vi "Read Application Settings.vi"(8 "error in":errorcluster, 11 "Controller in":refnum<class "Controller.lvclass">) -> (0 "error out":errorcluster, 2 "Application Settings":T4={"Storage Settings"={"Primary Path"=path "", "Backup Storage?"=FALSE, "Backup Path"=path "", "Component Name Prefix"="", "Image Format"=enum."<Select>"}, "PLC Settings"={"Port"="", "BaudRate"=9600, "Wakeup Signal Address "=0, "Acquisiton Address"=0, "Acknowledgement Address"=0, "Sleep Address"=0}, "Total Images"=0}, 3 "Controller out":refnum<class "Controller.lvclass">)   [LabVIEW 2021, in "Controller.lvlib" / "Controller.lvclass"]
uses:
  Controller.lvclass
  <vilib>/Utility/config.llb/NI_LVConfig.lvlib
  <vilib>/Utility/config.llb/Read Key (Path).vi
  <vilib>/Utility/config.llb/Read Key (String).vi
  <vilib>/Utility/config.llb/Read Key (U32).vi
  <vilib>/Utility/config.llb/Read Key (Boolean).vi
  Typedefs/Image Formats.ctl
  Typedefs/Storage Settings.ctl
  Typedefs/PLC Settings.ctl
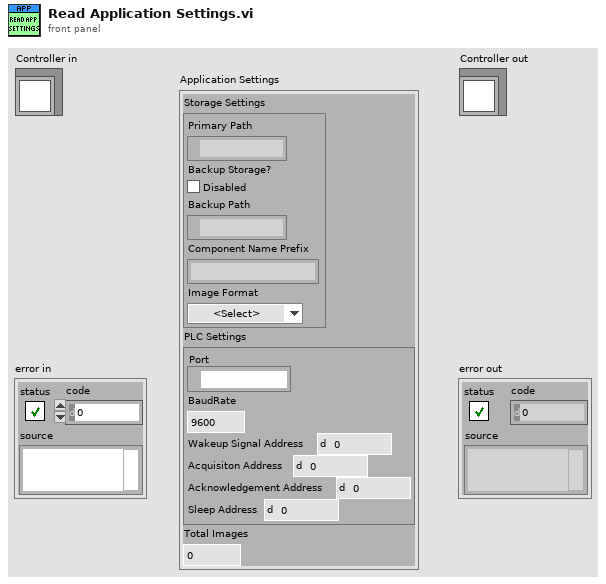
[diagram p1: front panel]
types:
  T1 = typedef "Storage Settings.ctl" = cluster{"Primary Path":path, "Backup Storage?":bool, "Backup Path":path, "Component Name Prefix":string, "Image Format":T2}
  T2 = typedef "Image Formats.ctl" = enum16{"<Select>", "TIFF", "RAW"}
  T3 = typedef "PLC Settings.ctl" = cluster{"Port":refnum<visa-resource-name>, "BaudRate":u32, "Wakeup Signal Address ":u16, "Acquisiton Address":u16, "Acknowledgement Address":u16, "Sleep Address":u16}
  T4 = cluster{"Storage Settings":T1, "PLC Settings":T3, "Total Images":u32}
  T5 = cluster{"Config File ":path, "Configuration":path, "Event Log":path, "Error Log":path}
  T6 = typedef "NI_LVConfig.lvlib/Config Data RefNum.ctl" = refnum<k1>
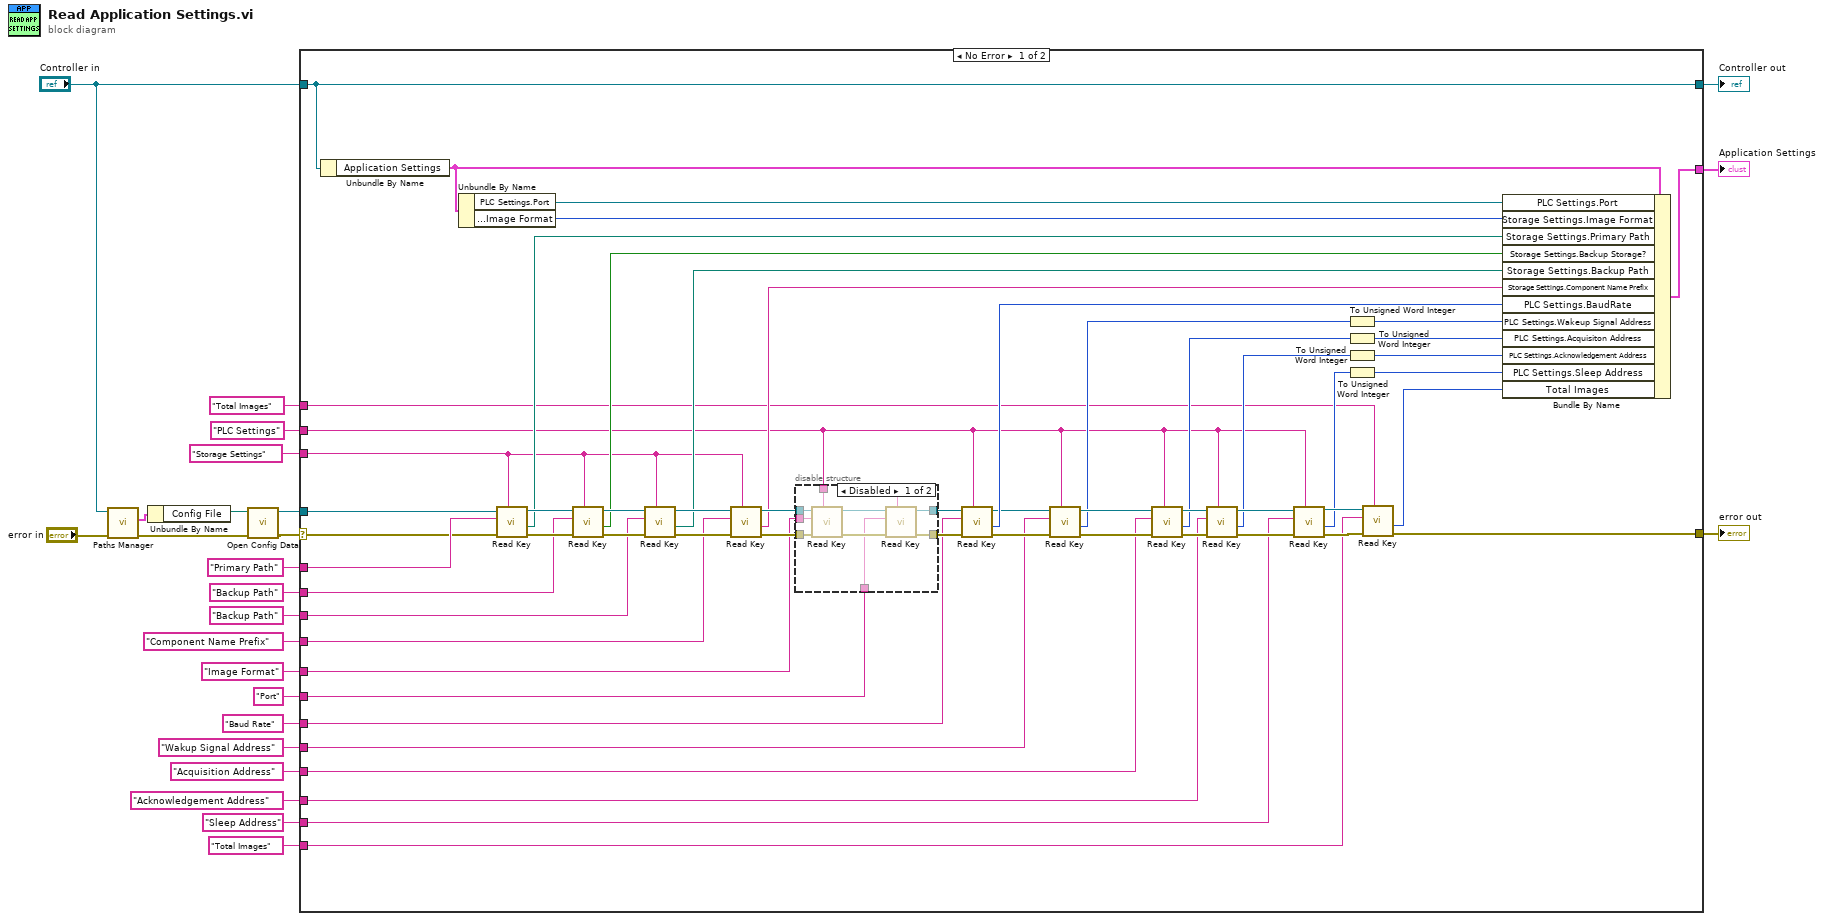
[diagram p0: block diagram]
diagram:
  n1 = call "Paths Manager.vi"("error in"="error in", "Controller in"="Controller in") -> ("error out"=w5:errorcluster, "Paths"=w4:T5)  [unwired: 7 in, 1 out]
  n2 = Unbundle By Name(w4) -> ("Config File"=w2:path)
  n3 = call <vilib>:"Open Config Data.vi"("error in (no error)"=w5, "configuration file path"=w2) -> ("error out"=w1:errorcluster, "refnum"=w7:T6)  [unwired: 7 in, 1 out]
  n4 = case shown="No Error" w1 {
    selector: w1 -> [w26 w94]
    tunnel: [w27 w94] -> w25
    tunnel: [w46 w95] -> w24
    tunnel: "Controller in" -> [w46 w95]
    tunnel: [w28 _] -> w23
    tunnel: "Total Images" -> [w44 _]
    tunnel: "PLC Settings" -> [w43 _]
    tunnel: "Storage Settings" -> [w42 _]
    tunnel: "Primary Path" -> [w41 _]
    tunnel: "Backup Path" -> [w40 _]
    tunnel: "Backup Path" -> [w39 _]
    tunnel: "Component Name Prefix" -> [w38 _]
    tunnel: "Image Format" -> [w37 _]
    tunnel: "Port" -> [w36 _]
    tunnel: "Baud Rate" -> [w35 _]
    tunnel: "Wakup Signal Address" -> [w34 _]
    tunnel: "Acquisition Address" -> [w33 _]
    tunnel: "Acknowledgement Address" -> [w32 _]
    tunnel: "Sleep Address" -> [w31 _]
    tunnel: "Total Images" -> [w30 _]
    tunnel: w7 -> [w29 _]
    frame No Error {
      n5 = Unbundle By Name(w46) -> ("Application Settings"=w45:T4)
      n6 = Unbundle By Name(w45) -> ("PLC Settings.Port"=w47:refnum<visa-resource-name>, "Storage Settings.Image Format"=w48:T2)
      n7 = call-poly <vilib>:"Read Key.vi"("section"=w42, "error in (no error)"=w26, "key"=w41, "refnum"=w29) -> ("error out"=w73:errorcluster, "value"=w60:path, "refnum out"=w66:T6)  [unwired: 4 in, 1 out]
      n8 = call-poly <vilib>:"Read Key.vi"("section"=w42, "error in (no error)"=w73, "key"=w40, "refnum"=w66) -> ("error out"=w82:errorcluster, "value"=w59:bool, "refnum out"=w65:T6)  [unwired: 4 in, 1 out]
      n9 = call-poly <vilib>:"Read Key.vi"("section"=w42, "error in (no error)"=w82, "key"=w39, "refnum"=w65) -> ("error out"=w81:errorcluster, "value"=w58:path, "refnum out"=w64:T6)  [unwired: 4 in, 1 out]
      n10 = call-poly <vilib>:"Read Key.vi"("section"=w42, "error in (no error)"=w81, "key"=w38, "refnum"=w64) -> ("error out"=w80:errorcluster, "value"=w57:string, "refnum out"=w63:T6)  [unwired: 4 in, 1 out]
      n11 = disable-structure shown="Disabled" {
        disable-tunnel: w80 -> [w91 w93]
        disable-tunnel: [w90 w93] -> w74
        disable-tunnel: w43 -> [w88 _]
        disable-tunnel: w63 -> [w87 w92]
        disable-tunnel: [w85 w92] -> w62
        disable-tunnel: w37 -> [w84 _]
        disable-tunnel: w36 -> [w83 _]
        frame Disabled {
          n12 = call-poly <vilib>:"Read Key.vi"("section"=w88, "error in (no error)"=w91, "key"=w84, "refnum"=w87) -> ("error out"=w89:errorcluster, "refnum out"=w86:T6)  [unwired: 4 in, 2 out]
          n13 = call-poly <vilib>:"Read Key.vi"("section"=w88, "error in (no error)"=w89, "key"=w83, "refnum"=w86) -> ("error out"=w90:errorcluster, "refnum out"=w85:T6)  [unwired: 4 in, 2 out]
        }
        frame Enabled {
        }
      }
      n14 = call-poly <vilib>:"Read Key.vi"("section"=w43, "error in (no error)"=w74, "key"=w35, "refnum"=w62) -> ("error out"=w79:errorcluster, "value"=w72:u32, "refnum out"=w61:T6)  [unwired: 4 in, 1 out]
      n15 = call-poly <vilib>:"Read Key.vi"("section"=w43, "error in (no error)"=w79, "key"=w34, "refnum"=w61) -> ("error out"=w78:errorcluster, "value"=w54:u32, "refnum out"=w67:T6)  [unwired: 4 in, 1 out]
      n16 = call-poly <vilib>:"Read Key.vi"("section"=w43, "error in (no error)"=w78, "key"=w33, "refnum"=w67) -> ("error out"=w77:errorcluster, "value"=w52:u32, "refnum out"=w68:T6)  [unwired: 4 in, 1 out]
      n17 = call-poly <vilib>:"Read Key.vi"("section"=w43, "error in (no error)"=w77, "key"=w32, "refnum"=w68) -> ("error out"=w76:errorcluster, "value"=w56:u32, "refnum out"=w69:T6)  [unwired: 4 in, 1 out]
      n18 = call-poly <vilib>:"Read Key.vi"("section"=w43, "error in (no error)"=w76, "key"=w31, "refnum"=w69) -> ("error out"=w75:errorcluster, "value"=w55:u32, "refnum out"=w70:T6)  [unwired: 4 in, 1 out]
      n19 = To Unsigned Word Integer(number=w54) -> (unsigned 16bit integer=w53:u16)
      n20 = To Unsigned Word Integer(number=w52) -> (unsigned 16bit integer=w51:u16)
      n21 = To Unsigned Word Integer(number=w56) -> (unsigned 16bit integer=w50:u16)
      n22 = To Unsigned Word Integer(number=w55) -> (unsigned 16bit integer=w49:u16)
      n23 = call-poly <vilib>:"Read Key.vi"("section"=w44, "error in (no error)"=w75, "key"=w30, "refnum"=w70) -> ("error out"=w27:errorcluster, "value"=w71:u32)  [unwired: 4 in, 2 out]
      n24 = Bundle By Name(cluster=w45, "PLC Settings.Port"=w47, "Storage Settings.Image Format"=w48, "Storage Settings.Primary Path"=w60, "Storage Settings.Backup Storage?"=w59, "Storage Settings.Backup Path"=w58, "Storage Settings.Component Name Prefix"=w57, "PLC Settings.BaudRate"=w72, "PLC Settings.Wakeup Signal Address"=w53, "PLC Settings.Acquisiton Address"=w51, "PLC Settings.Acknowledgement Address"=w50, "PLC Settings.Sleep Address"=w49, "Total Images"=w71) -> (w28:T4)
    }
    frame Error {
    }
  }
  "error out" <- w25
  "Controller out" <- w24
  "Application Settings" <- w23
